vi "System Information.vi"() -> (0 "Memory Statistics":T1 {"Available Virtual Memory (MB)" format="%.2f"; "Total Virtual Memory (MB)" format="%.2f"; "Available Page File (MB)" format="%.6f"; "Total Page File (MB)" format="%.2f"; "Available Physical Memory (MB)" format="%.2f"; "Total Physical Memory (MB)" format="%.2f"; "% mem used" format="%.2f"}, 1 "system information":T2 {"is NT?" format="%.2f"; "Windows Version" format="%.2f"})   [LabVIEW 2013]
doc: "This VI retrieves information about the computer system and operating environment.\n\nWin32\n======\n% free resources information is not returned, and presence of a coprocessor may not be correctly reported on 80386 machines. 386Enh and virtual memory are always in effect. More memory information is available in the Memory Statistics cluster."
uses:
  kernel32.dll
  LVWUtil32.dll
panel:
  out "processor":u8(ring) items=["Unknown", "Intel 386", "Intel 486", "Pentium"]
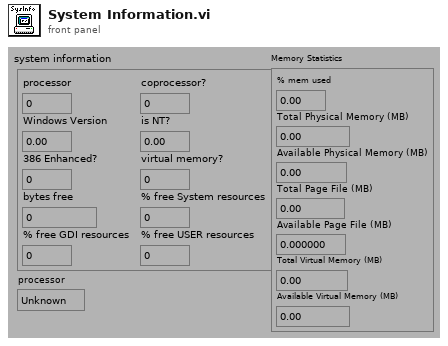
[diagram p1: front panel]
types:
  T1 = cluster{"% mem used":dbl, "Total Physical Memory (MB)":dbl, "Available Physical Memory (MB)":dbl, "Total Page File (MB)":dbl, "Available Page File (MB)":dbl, "Total Virtual Memory (MB)":dbl, "Available Virtual Memory (MB)":dbl}
  T2 = cluster{"processor":u32, "coprocessor?":u32, "Windows Version":sgl, "is NT?":sgl, "386 Enhanced?":u32, "virtual memory?":u32, "bytes free":u32, "% free System resources":u32, "% free GDI resources":u32, "% free USER resources":u32}
  T3 = cluster{"% mem used":u32, "Total Physical Memory":u32, "Available Physical Memory":u32, "Total Page File":u32, "Available Page File":u32, "Total Virtual Memory":u32, "Available Virtual Memory":u32}
  T4 = cluster{"[0]":dbl, "[1]":dbl, "[2]":dbl, "[3]":dbl, "[4]":dbl, "[5]":dbl, "[6]":dbl}
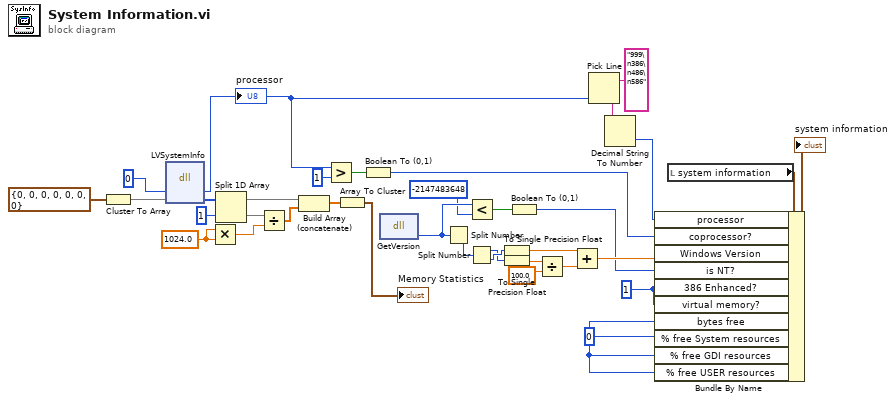
[diagram p0: block diagram]
diagram:
  w10 = u32 1 ("386 Enhanced?")
  w12 = 1024.0
  w11 = u32 0 ("% free System resources")
  n1 = Cluster To Array(cluster=T3 {"% mem used"=0, "Total Physical Memory"=0, "Available Physical Memory"=0, "Total Page File"=0, "Available Page File"=0, "Total Virtual Memory"=0, "Available Virtual Memory"=0} ("Memory Statistics")) -> (array=w21:u32[])
  n2 = dll-call lib="C:/Users/HamiltonDesignAir/Documents/~LabVIEW Archive/LabVIEW Programming Resource/WIN Event/lvwutil32.dll" fn="LVSystemInfo"("dwProcessorType"=u8 0 ("processor"), "lvMemStats"=w21) -> ("dwProcessorType"=w6:u8, "lvMemStats"=w19:u32[])  [unwired: 4 in, 2 out]
  "processor" <- w6
  n3 = Multiply(x=w12, y=w12) -> (x*y=w13:dbl)
  n4 = Split 1D Array(array=w19, index=1) -> (first subarray=w17:u32[], second subarray=w15:u32[])
  n5 = Divide(x=w15, y=w13) -> (x/y=w16:dbl[])
  n6 = Build Array (concatenate)(w17, w16) -> (w14:dbl[])
  n7 = Greater?(x=w6, y=u8 1) -> (0:w8:bool)
  n8 = Array To Cluster(array=w14) -> (cluster=→"Memory Statistics":T4)
  n9 = Boolean To (0,1)(Boolean=w8) -> (0, 1=w7:i16)
  n10 = dll-call lib="kernel32.dll" fn="GetVersion"() -> ("Versions"=w4:u32)  [unwired: 3 in, 2 out]
  n11 = Split Number(x=w4) -> (lo(x)=w29:u16)  [unwired: 1 out]
  n12 = Less?(x=w4, y=-2147483648) -> (x < y?=w2:bool)
  n13 = Split Number(x=w29) -> (hi(x)=w34:u8, lo(x)=w35:u8)
  n14 = To Single Precision Float(number=w35) -> (single precision float=w30:sgl)
  n15 = To Single Precision Float(number=w34) -> (single precision float=w33:sgl)
  n16 = Boolean To (0,1)(Boolean=w2) -> (0, 1=w1:i16)
  n17 = Divide(x=w33, y=sgl 100.0) -> (x/y=w31:sgl)
  n18 = Add(x=w30, y=w31) -> (x+y=w28:sgl)
  n19 = Pick Line(multi-line string="999\n386\n486\n586", line index=w6) -> (output string=w24:string)  [unwired: 1 in]
  n20 = Decimal String To Number(string=w24) -> (number=w23:i32)  [unwired: 2 in, 1 out]
  n21 = local read "system information"() -> (w27:T2)
  n22 = Bundle By Name(cluster=w27, "processor"=w23, "coprocessor?"=w7, "Windows Version"=w28, "is NT?"=w1, "386 Enhanced?"=w10, "virtual memory?"=w10, "bytes free"=w11, "% free System resources"=w11, "% free GDI resources"=w11, "% free USER resources"=w11) -> (→"system information":T2)
